vi "Save Xml in DOM(traverse).vi"(8 "error in":errorcluster caption="错误输入（无错误）", 10 "Data in":T1, 11 "PanelRootNode.lvclass":refnum<class "PanelRootNode.lvclass">) -> (0 "error out":errorcluster caption="错误输出", 2 "Data out":T1, 3 "PanelRootNode out":refnum<class "PanelRootNode.lvclass">)   [LabVIEW 2016, in "PanelRootNode.lvclass"]
uses:
  PanelRootNode.lvclass
  C:/Users/CL/Desktop/ZcDAQprj0811/ZcDAQprj/Modules/DAQ-Display/PanelSplitToolkit/PanelLinkNode/PanelLinkNode.lvclass
  PanelLinkNode/PanelLinkNode.lvclass/PanelLinkNode.ctl
  <vilib>/xml/Close Reference(Node).vi
  PanelObject/PanelObject.lvclass
  PanelLinkNode/PanelLinkNode.lvclass
  <vilib>/xml/NI_XML.lvlib
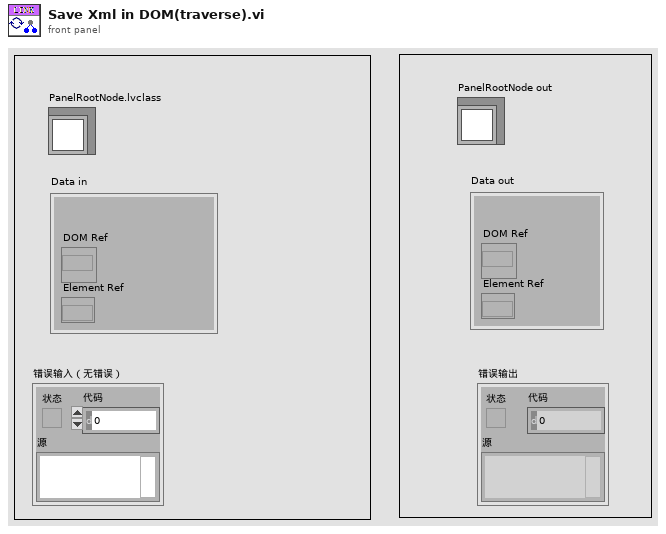
[diagram p1: front panel]
types:
  T1 = cluster{"DOM Ref":refnum<k20>, "Element Ref":refnum<k20>}
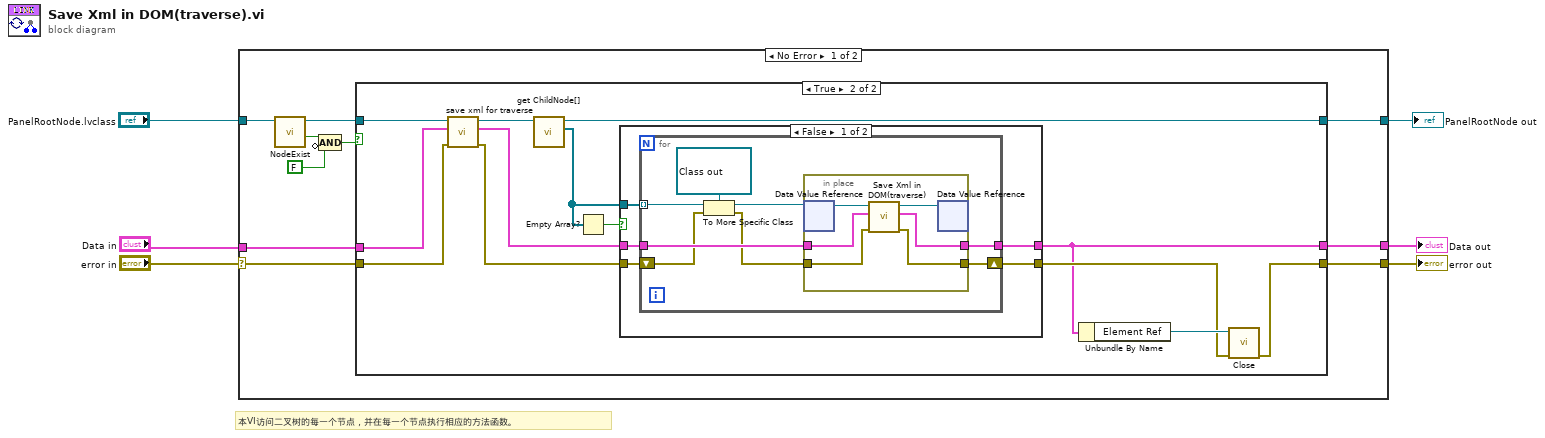
[diagram p0: block diagram]
diagram:
  # "本VI访问二叉树的每一个节点，并在每一个节点执行相应的方法函数。"
  n1 = case shown="No Error" "error in" {
    selector: "error in" -> [w8 w56]
    tunnel: [w12 w56] -> w5
    tunnel: [w16 w55] -> w3
    tunnel: "PanelRootNode.lvclass" -> [w15 w55]
    tunnel: [w13 w54] -> w1
    tunnel: "Data in" -> [w9 w54]
    frame No Error {
      n2 = call-dynamic "NodeExist.vi"("PanelLinkNode 输入"=w15) -> ("Node Exist?"=w11:bool, "PanelLinkNode 输出"=w14:refnum<class "PanelRootNode.lvclass">)  [unwired: 8 in, 1 out]
      n3 = Compound Arithmetic op=AND(w11, invert FALSE ("值")) -> (w10:bool)
      n4 = case shown="True" w10 {
        tunnel: [w19 w32] -> w16
        tunnel: w14 -> [w19 w31]
        tunnel: [w17 w20] -> w13
        tunnel: [w18 w23] -> w12
        tunnel: w8 -> [w18 w28]
        tunnel: w9 -> [w17 w29]
        frame False {
        }
        frame True {
          n5 = call-dynamic "save xml for traverse.vi"("error in"=w28, "Data in"=w29, "PanelRootNode 输入"=w31) -> ("error out"=w27:errorcluster, "Data out"=w26:T1, "PanelRootNode 输出"=w30:refnum<class "PanelRootNode.lvclass">)  [unwired: 6 in]
          n6 = call "get ChildNode[].vi"("PanelLinkNode输入"=w30) -> ("ChildNode*[]"=w22:refnum<data-value>[], "PanelLinkNode输出"=w32:refnum<class "PanelRootNode.lvclass">)  [unwired: 8 in, 1 out]
          n7 = Empty Array?(array=w22) -> (empty?=w21:bool)
          n8 = case shown="False" w21 {
            tunnel: [w37 w53] -> w20
            tunnel: w22 -> [w36 _]
            tunnel: w27 -> [w35 w52]
            tunnel: w26 -> [w34 w53]
            tunnel: [w33 w52] -> w24
            frame False {
              n9 = for {
                tunnel: w36 -> [w45] mode=indexing
                shift-right: [w42] -> w33
                shift-left: w35 -> [w40]
                tunnel: w34 -> [w43]
                tunnel: [w41] -> w37
                n10 = To More Specific Class(target class=refnum<data-value> refnum ("数据值引用"), reference=w45, error in=w40) -> (specific class reference=w44:refnum<data-value>, error out=w39:errorcluster)
                n11 = in-place {
                  in-place-border: w43 -> [w48]
                  in-place-border: w39 -> [w47]
                  in-place-border: [w46] -> w42
                  in-place-border: [w49] -> w41
                  n12 = in-place-dvr #1(w44) -> (w51:refnum<class "PanelRootNode.lvclass">)  [unwired: 1 out]
                  n13 = call "Save Xml in DOM(traverse).vi"("error in"=w47, "Data in"=w48, "PanelRootNode.lvclass"=w51) -> ("error out"=w46:errorcluster, "Data out"=w49:T1, "PanelRootNode out"=w50:refnum<class "PanelRootNode.lvclass">)  [unwired: 6 in]
                  n14 = in-place-dvr #1(w50) -> ()  [unwired: 2 out]
                }
              }
            }
            frame True {
            }
          }
          n15 = Unbundle By Name(w20) -> ("Element Ref"=w25:refnum<k20>)
          n16 = call-poly <vilib>:"Close.vi"("error in (no error)"=w24, "node"=w25) -> ("error out"=w23:errorcluster)  [unwired: 7 in]
        }
      }
    }
    frame Error {
    }
  }
  "error out" <- w5
  "PanelRootNode out" <- w3
  "Data out" <- w1
